vi "[Property] Cursor Pairs Write.vi"(4 "error in (no error)":errorcluster, 5 "Value":u32, 6 "Container State":T2, 7 "Display State In":T1) -> (0 "error out":errorcluster, 3 "Display State Out":T1)   [LabVIEW 2014, in "Graph with cursors XControl.xctl"]
uses:
  Graph with cursors XControl.xctl
  <vilib>/_xctls/Container State.ctl
  Graph with cursors State.ctl
  <vilib>/_xctls/XControlSupport.lvlib
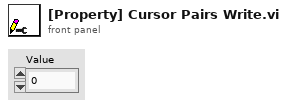
[diagram p1: front panel]
types:
  T1 = typedef "Graph with cursors XControl.xctl/Graph with cursors State.ctl" = cluster{"Cursor names":string[], "Cursor positions":dbl[], "Cursor pairs":i32, "Graph":refnum<vi>, "Prefix":string, "Base path":path}
  T2 = typedef "XControlSupport.lvlib/Container State.ctl" = cluster{"Indicator?":bool, "Run Mode?":bool, " Refnum":refnum<vi>}
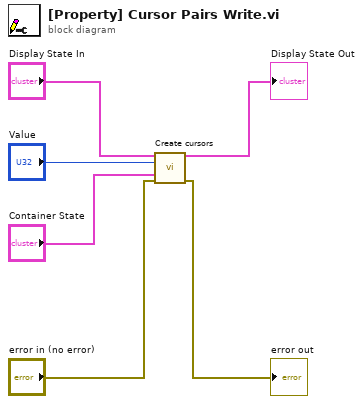
[diagram p0: block diagram]
diagram:
  n1 = call "Create cursors.vi"("Display State In"="Display State In", "Cursor pairs"="Value", "Container State"="Container State", "error in (no error)"="error in (no error)") -> ("Display State Out"=→"Display State Out":T1, "error out"=→"error out":errorcluster)  [unwired: 10 in]
